vi "Drive with Angle.vi"(6 "Synchronization":enum16{"Start", "Wait"}(ring), 7 "Description":string, 8 "Command Info In":T1, 9 "Angle Icrement":dbl, 10 "Straight Speed":dbl) -> (0 "Command Info Out":T1, 3 "Outcome":string="foo")   [LabVIEW 2016]
doc: "This VI sets the motors to run for a given number of seconds. It optionally synchronizes with the completion of the command."
uses:
  <vilib>/Rock Robotics/WPI/Framework/Command Status Info.ctl
  <vilib>/Rock Robotics/WPI/Framework/Completion Status.ctl
  <vilib>/Rock Robotics/WPI/Framework/Completion Notifier.ctl
  Implementation/Drive Setpoints.ctl
  Implementation/Drive Operations.ctl
panel:
  in  "Deadband Angle":dbl=1.0
  in  "Deadband Value":dbl=0.01
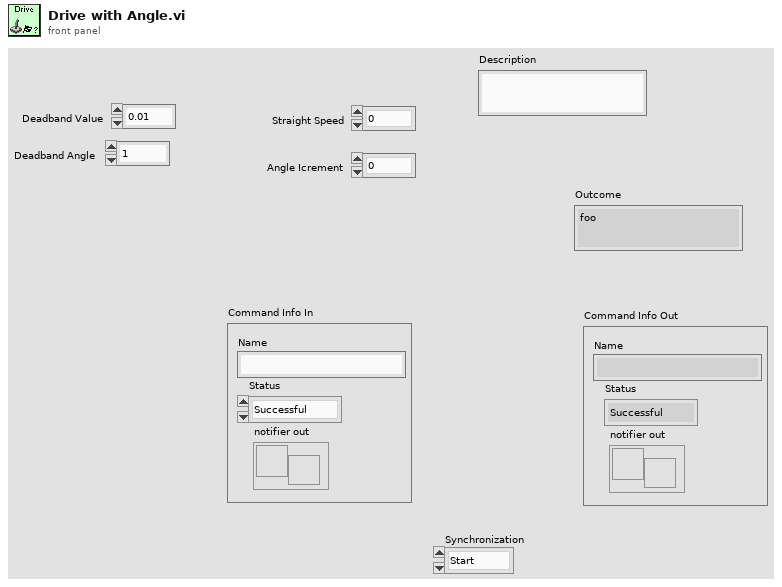
[diagram p1: front panel]
types:
  T1 = typedef "Command Status Info.ctl" = cluster{"Name":string, "Status":T2, "notifier out":T3}
  T2 = typedef "Completion Status.ctl" = enum16{"Successful", "Aborted", "Incomplete"}
  T3 = typedef "Completion Notifier.ctl" = refnum<notifier>
  T4 = typedef "Drive Setpoints.ctl" = cluster{"Operation":T5, "Left Setpoint":dbl, "Right Setpoint":dbl, "Duration":dbl}
  T5 = typedef "Drive Operations.ctl" = enum16{"Reserve", "Read Current", "Immediate", "Drive for Time", "Drive for Distance", "Drive for Angle", "Drive with Angle"}
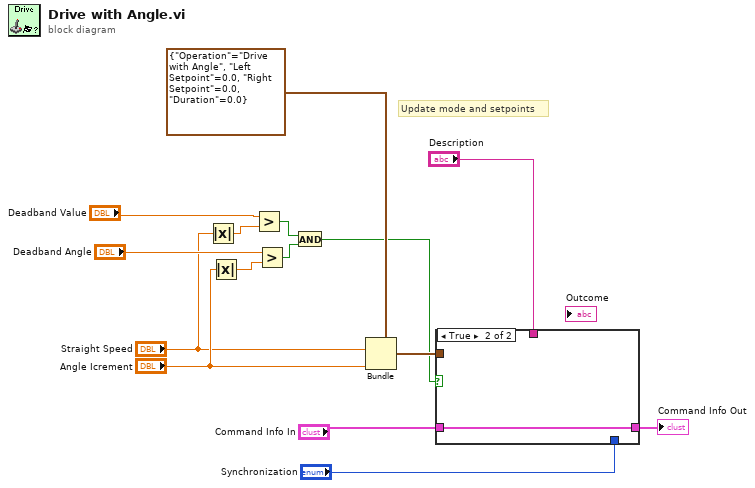
[diagram p0: block diagram]
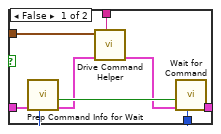
[diagram p2: hidden frame]
diagram:
  # "Update mode and setpoints"
  n1 = Absolute Value(x="Straight Speed") -> (abs(x)=w9:dbl)
  n2 = Absolute Value(x="Angle Icrement") -> (abs(x)=w7:dbl)
  n3 = Greater?(x="Deadband Value", y=w9) -> (0:w8:bool)
  n4 = Greater?(x="Deadband Angle", y=w7) -> (0:w6:bool)
  n5 = And(x=w8, y=w6) -> (x .and. y?=w1:bool)
  n6 = Bundle(cluster=T4 {"Operation"=enum."Drive with Angle", "Left Setpoint"=0.0, "Right Setpoint"=0.0, "Duration"=0.0} ("SubSystem Data"), "Left Setpoint"="Straight Speed", "Duration"="Angle Icrement") -> (w11:T4)  [unwired: 2 in]
  n7 = case shown="True" w1 {
    tunnel: "Description" -> [w23 _]
    tunnel: "Command Info In" -> [w20 w24]
    tunnel: [w19 w24] -> w12
    tunnel: w11 -> [w17 _]
    tunnel: "Synchronization" -> [w16 _]
    frame False {
      n8 = call <vilib>:"Prep Command Info for Wait.vi"("Synchronication"=w16, "Command Info"=w20) -> ("Command Info"=w21:T1, "Allocated"=w22:bool)  [unwired: 8 in]
      n9 = call "Drive Command Helper.vi"("Description"=w23, "Command Info In"=w21, "SubSystem Data"=w17) -> ("Command Info Out"=w18:T1)  [unwired: 7 in, 1 out]
      n10 = call <vilib>:"Wait for Command.vi"("Synchronication"=w16, "Command Info in"=w18, "Allocated"=w22) -> ("Command Info out"=w19:T1)  [unwired: 8 in]
    }
    frame True {
    }
  }
  "Command Info Out" <- w12
